vi "ReadHoldingRegisters.vi"   [LabVIEW 2018]
uses:
  <vilib>/Plasmionique/MB Master/MB_Master/MB_Master.lvclass
  <vilib>/Plasmionique/MB Master/MB Master.lvlib
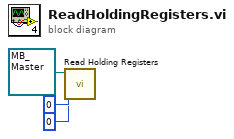
[diagram p0: block diagram]
diagram:
  n1 = call <vilib>:"Read Holding Registers.vi"("quantity"=u16 0, "starting address"=u16 0, "MB session in"=refnum<class "MB_Master.lvclass"> refnum) -> ()  [unwired: 6 in, 3 out]
